vi "Load and decimate relevant raw data.vi"(8 "error in (no error)":errorcluster) -> (0 "error out":errorcluster, 1 "Data reference":refnum<data-value>, 2 "Total # of loaded points":i32, 3 "X-axis max/min (across all loaded data types)":cluster{"X-axis max":dbl, "X-axis min":dbl})   [LabVIEW 2017]
uses:
  xcontrol/Interface VIs/Interface typedefs/Interface-Data array.ctl
  xcontrol/Interface VIs/Interface typedefs/Interface-Data format definition.ctl
  xcontrol/Typedefs/Xctl-XY data type definition.ctl
  xcontrol/Typedefs/Xctrl-ROI type enum.ctl
  Global variables/gl_Functional Imaging-Global variables.vi
  xcontrol/XGrapher.xctl
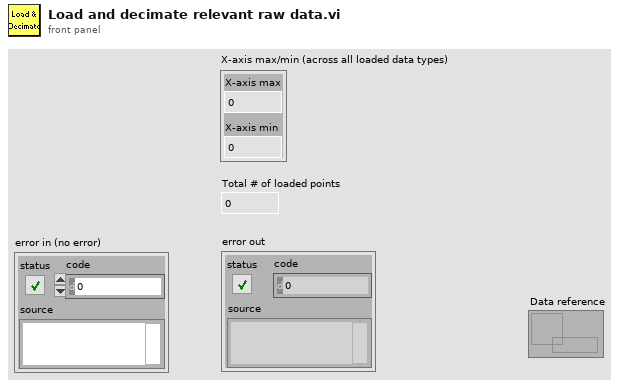
[diagram p1: front panel]
types:
  T1 = typedef "Functional Imging UI Refs.ctl" = cluster{"Menu ref":refnum<k9>, "Image control":refnum<vi>, "VI ref":refnum<vi>, "XGrapher":refnum<vi>, "Smoothing":refnum<vi>, "POI Averaging":refnum<vi>, "Normalize":refnum<vi>, "POI data points in each trial":refnum<vi>, "Channel":refnum<vi>, "Experiment data folder path":refnum<vi>, "[ROI vis]":refnum<vi>, "[Groups] visbl":T2, "Group Name":refnum<vi>, "POI index":refnum<vi>, "Trial No.":refnum<vi>, "Intensity Zoom":refnum<vi>, "Trial Cursor Enabled":refnum<vi>, "Number of Trials (ind 1)":refnum<vi>, "Number of Trials (ind 2)":refnum<vi>, "MiniScans Available":refnum<vi>, "POI Available":refnum<vi>, "Defer graph updates":refnum<vi>, "Waveform selector":refnum<vi>, "#of selected POI":refnum<vi>, "#of selected MiniScans":refnum<vi>, "#of selected groups":refnum<vi>, "Max Z-Projection":refnum<vi>, "Z-Plane Selector":refnum<vi>, "Index of miniscan point to visualise":refnum<vi>, "ROI vis. mode":refnum<vi>, "Total # of points":refnum<vi>, "Index of group clicked on":refnum<vi>, "Pane 1":refnum<vi>, "Pane 2":refnum<vi>, "Pane 3":refnum<vi>, "Pane 4":refnum<vi>, "Pane 5":refnum<vi>, "Pane 6":refnum<vi>, "Deselect all ROI":refnum<vi>, "Deselect all groups":refnum<vi>}
  T2 = typedef "Groups array referecne.ctl" = refnum<vi>
  T3 = typedef "Interface-Data array.ctl" = T4[]
  T4 = typedef "Interface-Data format definition.ctl" = cluster{"Plot.Plot Name":string, "Data":T5, "Timeline data":T5, "Type":T6, "Points per cycle":u16, "ROI number":u16}
  T5 = typedef "XGrapher.xctl/Xctl-XY data type definition.ctl" = cluster{"X-Axis values":sgl[], "Y-Axis values (s)":sgl[]}
  T6 = typedef "Xctrl-ROI type enum.ctl" = enum16{"POI", "Mini-scan", "Group"}
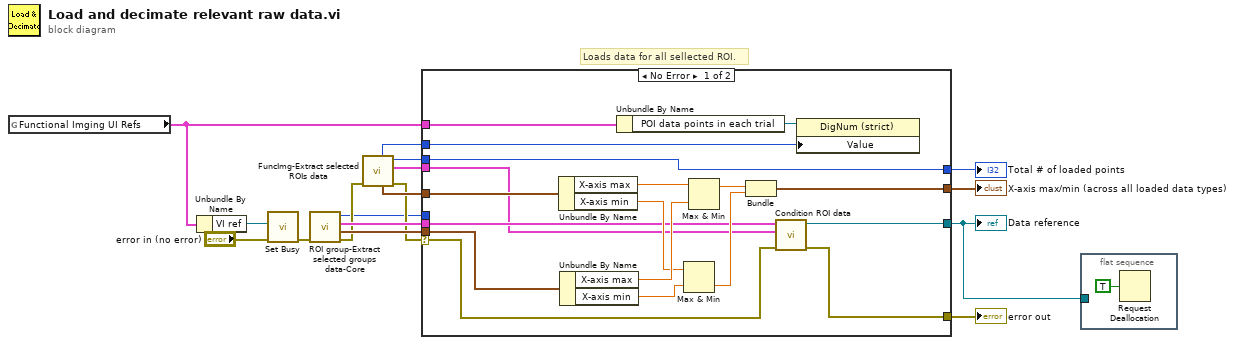
[diagram p0: block diagram]
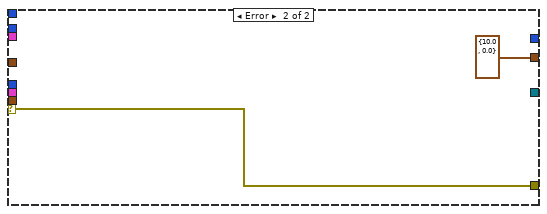
[diagram p2: hidden frame]
diagram:
  # "Loads data for all sellected ROI."
  n1 = global read "gl_Functional Imaging-Global variables.vi" "Functional Imging UI Refs"() -> (w3:T1)
  n2 = Unbundle By Name(w3) -> ("VI ref"=w2:refnum<vi>)
  n3 = call <vilib>:"Set Busy.vi"("error in (no error)"="error in (no error)", "VI reference (current VI)"=w2) -> ("error out"=w5:errorcluster)  [unwired: 8 in, 1 out]
  n4 = call "ROI group-Extract selected groups data-Core.vi"("error in"=w5) -> ("Error out"=w7:errorcluster, "X-axis max/min"=w13:cluster{"X-axis max":dbl, "X-axis min":dbl}, "Data for ticked Groups"=w14:T3, "Number of selected groups"=w1:i32)  [unwired: 7 in]
  n5 = call "FuncImg-Extract selected ROIs data.vi"("error in (no error)"=w7) -> ("error out"=w8:errorcluster, "Data for ticked ROI"=w10:T3, "Total number of points"=w11:i32, "X-axis max/min"=w9:cluster{"X-axis max":dbl, "X-axis min":dbl}, "Points in each trial"=w12:i32)  [unwired: 5 in, 1 out]
  n6 = case shown="No Error" w8 {
    selector: w8 -> [w21 w37]
    tunnel: [w22 w37] -> w17
    tunnel: [w25 _] -> w16
    tunnel: [w34 cluster{dbl, dbl} {10.0, 0.0}] -> w15
    tunnel: w14 -> [w19 _]
    tunnel: w13 -> [w27 _]
    tunnel: w12 -> [w26 _]
    tunnel: w11 -> [w25 _]
    tunnel: w10 -> [w18 _]
    tunnel: w9 -> [w24 _]
    tunnel: [w23 _] -> w6
    tunnel: w3 -> [w20 _]
    tunnel: w1 -> [_ _]
    frame No Error {
      n7 = Unbundle By Name(w24) -> ("X-axis max"=w33:dbl, "X-axis min"=w30:dbl)
      n8 = Unbundle By Name(w27) -> ("X-axis max"=w32:dbl, "X-axis min"=w29:dbl)
      n9 = Unbundle By Name(w20) -> ("POI data points in each trial"=w35:refnum<vi>)
      n10 = Max & Min(x=w30, y=w29) -> (min(x,y)=w28:dbl)  [unwired: 1 out]
      n11 = Max & Min(x=w33, y=w32) -> (max(x,y)=w31:dbl)  [unwired: 1 out]
      n12 = Bundle(w31, w28) -> (w34:cluster{dbl, dbl})  [unwired: 1 in]
      n13 = call "Condition ROI data.vi"("error in (no error)"=w21, "Data for ticked ROI"=w18, "Data for ticked Groups"=w19) -> ("error out"=w22:errorcluster, "Data reference"=w23:refnum<data-value>)  [unwired: 7 in]
      n14 = property class="DigNum (strict)"(reference=w35, "Value"=w26) -> ()  [unwired: 1 in, 2 out]
    }
    frame Error {
    }
  }
  "error out" <- w17
  "Total # of loaded points" <- w16
  "X-axis max/min (across all loaded data types)" <- w15
  "Data reference" <- w6
  n15 = flat-sequence {
    tunnel: w6 -> [_]
    frame #0 {
      n16 = Request Deallocation(TRUE ("flag")) -> ()
    }
  }
